vi "배열.vi"() -> ()   [LabVIEW 2014]
panel:
  in  "배열 2":dbl[](array[numeric])
  in  "배열":dbl[](array[numeric])=[0.0, 0.0, 0.0, 123.0]
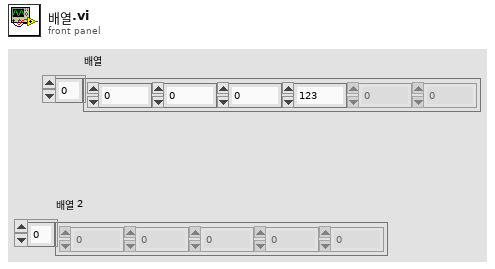
[diagram p1: front panel]
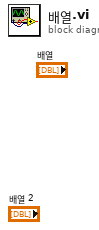
[diagram p0: block diagram]
diagram:
